vi "KG get mp sp.vi"(8 "Fehler (Eingang, kein Fehler)":errorcluster, 10 "pump":u32, 11 "VISA-Ressourcenname":refnum<visa-resource-name>) -> (0 "Fehler (Ausgang)":errorcluster, 1 "Kommando gesendeet":string, 2 "Flow":dbl, 3 "VISA-Ressourcenname (Ausgang)":refnum<visa-resource-name>)   [LabVIEW 2020, in "Linearisierung v2.lvlib" / "Gasteiler.lvlib" / "HovaCAL_Interface.lvlib" / "KGN.lvlib" / "get.lvlib"]
uses:
  get.lvlib
  KGN.lvlib
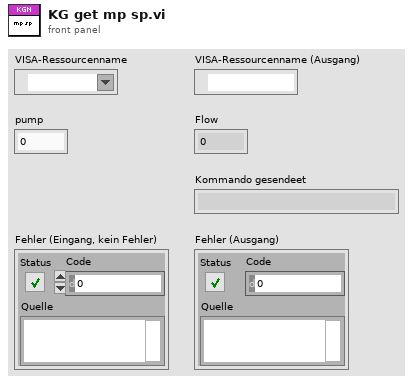
[diagram p1: front panel]
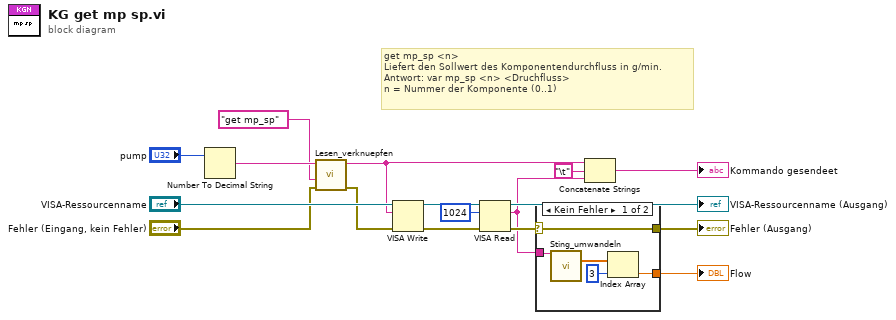
[diagram p0: block diagram]
diagram:
  # "get mp_sp <n>\nLiefert den Sollwert des Komponentendurchfluss in g/min.\nAntwort: var mp_sp <n> <Druchfluss>\nn = Nummer der Komponente (0..1)"
  n1 = Number To Decimal String(number="pump") -> (decimal integer string=w7:string)  [unwired: 1 in]
  n2 = call "Lesen_verknuepfen.vi"("error in (no error)"="Fehler (Eingang, kein Fehler)", "Order"="get mp_sp" ("Schreibpuffer"), "param"=w7) -> ("error out"=w9:errorcluster, "Verknüpfter String"=w8:string)  [unwired: 7 in]
  n3 = VISA Write(VISA resource name="VISA-Ressourcenname", write buffer=w8, error in (no error)=w9) -> (VISA resource name out=w17:refnum<visa-resource-name>, error out=w16:errorcluster)  [unwired: 1 out]
  n4 = VISA Read(VISA resource name=w17, byte count=u32 1024 ("Byte-Anzahl"), error in (no error)=w16) -> (VISA resource name out=→"VISA-Ressourcenname (Ausgang)":refnum<visa-resource-name>, read buffer=w2:string, error out=w5:errorcluster)  [unwired: 1 out]
  n5 = case shown="Kein Fehler" w5 {
    selector: w5 -> [w21 _]
    tunnel: w2 -> [w22 _]
    tunnel: [w18 _] -> w12
    tunnel: [w21 _] -> w4
    frame No Error {
      n6 = call "Sting_umwandeln.vi"("Lesepuffer"=w22) -> ("Zahl array"=w19:dbl[])  [unwired: 8 in, 6 out]
      n7 = Index Array(array=w19, index=3 ("Index")) -> (element=w18:dbl)
    }
    frame Error {
    }
  }
  "Fehler (Ausgang)" <- w4
  "Flow" <- w12
  n8 = Concatenate Strings(w8, "\t", w2) -> (→"Kommando gesendeet":string)
